vi "Serial Write Data.vi"(0 "VISA resource name":refnum<visa-resource-name>="COM1", 5 "trimmed string":string="0:0:0 UE 0 LE 0 COMP 0 FAN1 0 FAN2 0 SP:0 0 0 0 0 0 C030", 11 "error in (no error)":errorcluster) -> (15 "error out":errorcluster)   [LabVIEW 2009]
uses:
  <vilib>/Instr/_visa.llb/VISA Configure Serial Port (Instr).vi
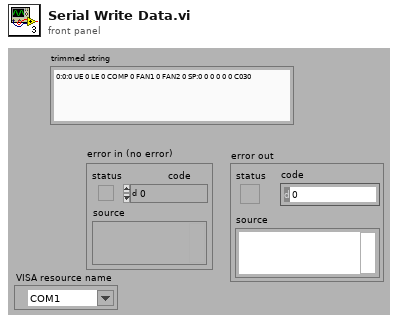
[diagram p1: front panel]
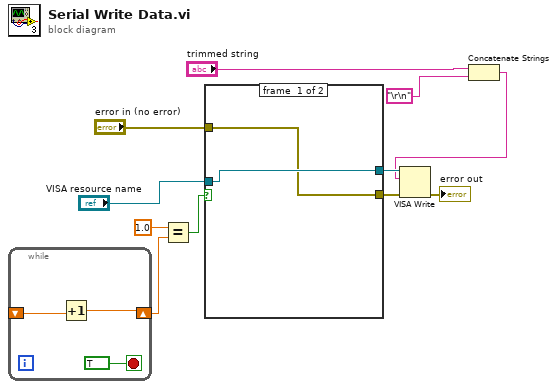
[diagram p0: block diagram]
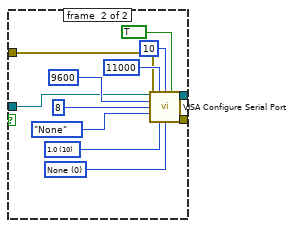
[diagram p2: hidden frame]
diagram:
  n1 = while {
    shift-right: [w12] -> w3
    shift-left: _ -> [w13]
    stop <- TRUE stop-if-true
    n2 = Increment(x=w13) -> (x+1=w12:dbl)
  }
  n3 = Equal?(x=1.0, y=w3) -> (x = y?=w1:bool)
  n4 = case shown="False" w1 {
    tunnel: "VISA resource name" -> [w16 w21]
    tunnel: [w16 w20] -> w10
    tunnel: "error in (no error)" -> [w15 w18]
    tunnel: [w15 w17] -> w4
    frame #0 {
    }
    frame #1 {
      w24 = u16 0 items=["None", "XON/XOFF", "RTS/CTS", "XON/XOFF & RTS/CTS", "DTR/DSR", "XON/XOFF & DTR/DSR"] ("flow control (0:none)")
      w25 = u16 10 items=["1.0"=10, "1.5"=15, "2.0"=20] ("stop bits (10: 1 bit)")
      n5 = call-poly "VISA Configure Serial Port"("VISA resource name"=w21, "timeout (10sec)"=u32 11000, "termination char\n(0xA = '\\n' = LF)"=u8 10 ("termination char\n(0xA = '\\n' = LF)"), "Enable Termination\nChar (T)"=TRUE ("Enable Termination\nChar (T)"), "baud rate (9600)"=u32 9600, "data bits (8)"=u16 8, "parity (0:none)"=enum16{"None", "Odd", "Even", "Mark", "Space"}."None", "error in (no error)"=w18, "stop bits (10: 1 bit)"=w25, "flow control (0:none)"=w24) -> ("VISA resource name out"=w20:refnum<visa-resource-name>, "error out"=w17:errorcluster)  [unwired: 4 in]
    }
  }
  n6 = Concatenate Strings("trimmed string", "\r\n") -> (w7:string)
  n7 = VISA Write(VISA resource name=w10, write buffer=w7, error in (no error)=w4) -> (error out=→"error out":errorcluster)  [unwired: 2 out]
